vi "01-Circulo.vi"() -> ()   [LabVIEW 2020]
panel:
  in  "Tab Control":enum32{"Ellipse Function"}(tab)
  out "Gráfica de un Círculo":cluster{dbl[], dbl[]}(graph)
  out "Functio Result":dbl[](array[numeric])
  in  "A":dbl
  in  "B":dbl
  in  "stop":bool
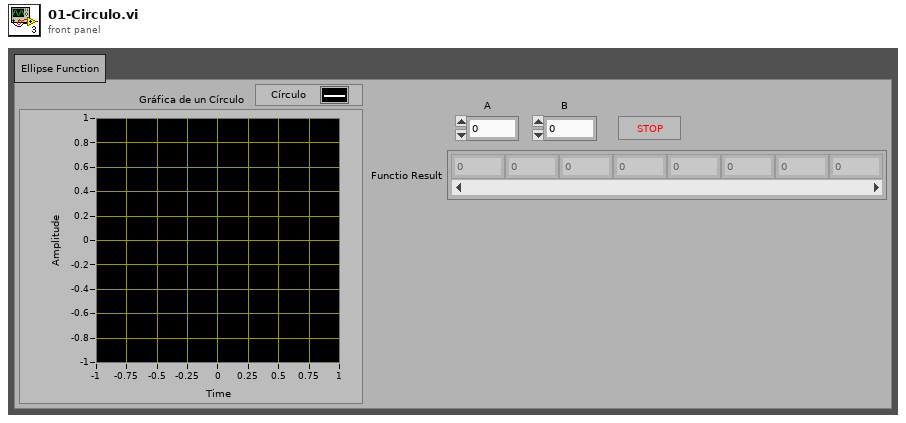
[diagram p1: front panel]
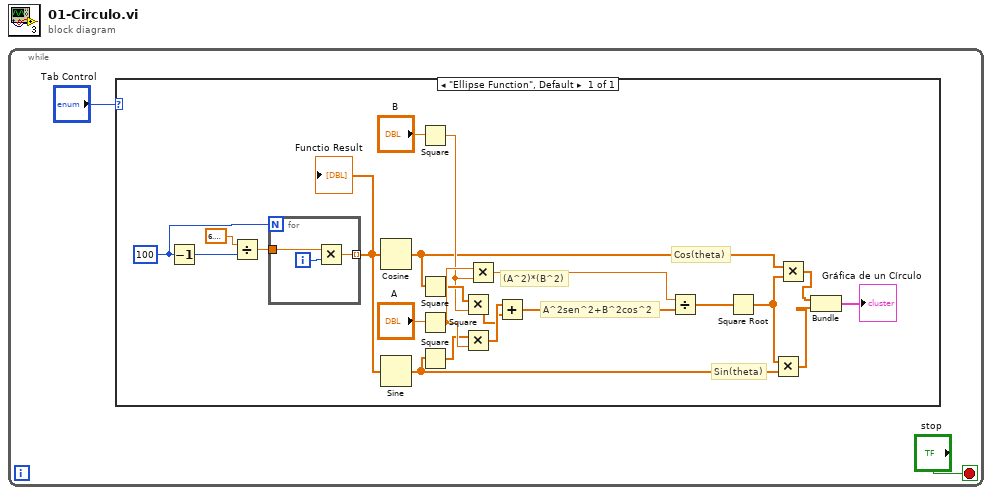
[diagram p0: block diagram]
diagram:
  n1 = while {
    stop <- "stop" stop-if-true
    n2 = case shown="\"Ellipse Function\", Default" "Tab Control" {
      frame "Ellipse Function", Default {
        w22 = 100
        # "Sin(theta)"
        # "Cos(theta)"
        # "A^2sen^2+B^2cos^2"
        # "(A^2)*(B^2)"
        n3 = Decrement(x=w22) -> (x-1=w24:i32)
        n4 = Divide(x=6.283185307179586, y=w24) -> (x/y=w21:dbl)
        n5 = for {
          N: w22 -> [_]
          tunnel: w21 -> [w27]
          tunnel: [w25] -> w20 mode=indexing
          i -> [w26]
          n6 = Multiply(x=w27, y=w26) -> (x*y=w25:dbl)
        }
        "Functio Result" <- w20
        n7 = Cosine(x=w20) -> (cos(x)=w8:dbl[])
        n8 = Sine(x=w20) -> (sin(x)=w7:dbl[])
        n9 = Square(x="B") -> (x^2=w16:dbl)
        n10 = Square(x=w8) -> (x^2=w17:dbl[])
        n11 = Square(x="A") -> (x^2=w19:dbl)
        n12 = Square(x=w7) -> (x^2=w18:dbl[])
        n13 = Multiply(x=w17, y=w16) -> (x*y=w3:dbl[])
        n14 = Multiply(x=w18, y=w19) -> (x*y=w4:dbl[])
        n15 = Multiply(x=w19, y=w16) -> (x*y=w15:dbl)
        n16 = Add(x=w4, y=w3) -> (x+y=w14:dbl[])
        n17 = Divide(x=w15, y=w14) -> (x/y=w13:dbl[])
        n18 = Square Root(x=w13) -> (sqrt(x)=w12:dbl[])
        n19 = Multiply(x=w12, y=w7) -> (x*y=w5:dbl[])
        n20 = Multiply(x=w8, y=w12) -> (x*y=w6:dbl[])
        n21 = Bundle(w6, w5) -> (→"Gráfica de un Círculo":cluster{dbl[], dbl[]})  [unwired: 1 in]
      }
    }
  }
